vi "TX.vi"(3 "error in (no error)":errorcluster, 4 "tx_buf":string, 5 "VISA resource name":refnum<visa-resource-name>="COM255") -> (0 "error out":errorcluster, 1 "envio OK":bool, 2 "VISA resource name OUT":refnum<visa-resource-name>)   [LabVIEW 2012]
panel:
  out "return count":u32
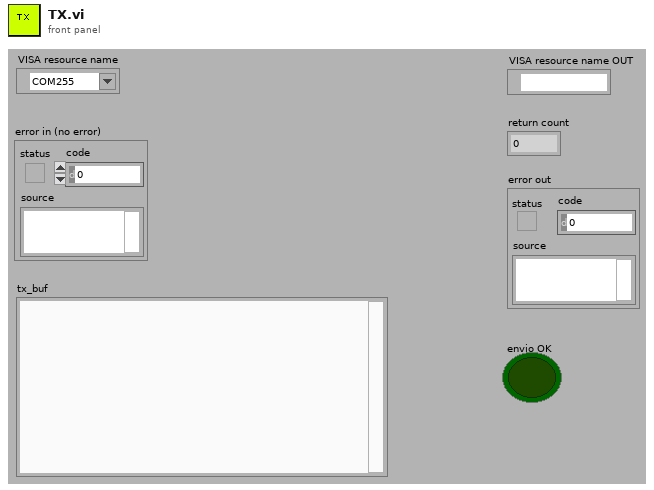
[diagram p1: front panel]
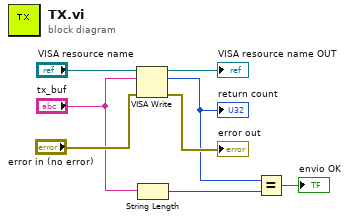
[diagram p0: block diagram]
diagram:
  n1 = VISA Write(VISA resource name="VISA resource name", write buffer="tx_buf", error in (no error)="error in (no error)") -> (VISA resource name out=→"VISA resource name OUT":refnum<visa-resource-name>, return count=w4:u32, error out=→"error out":errorcluster)
  "return count" <- w4
  n2 = String Length(string="tx_buf") -> (length=w3:i32)
  n3 = Equal?(x=w4, y=w3) -> (x = y?=→"envio OK":bool)
